vi "PH_Cam_BaseClass.set Cam Error.vi"(0 "VI in":refnum<vi>, 3 "Cam Error":errorcluster, 5 "error in":errorcluster) -> (14 "VI out":refnum<vi>, 19 "error out":errorcluster)   [LabVIEW 2014, in "PH_Cam_BaseClass.lvlib"]
doc: "This VI sets the Cam Error to own attributes and the GUI if it has changed."
uses:
  PH_Cam_BaseClass.lvlib
  PH_Common/PH_Common.lvlib
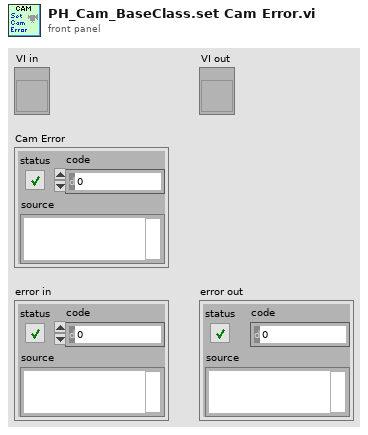
[diagram p1: front panel]
types:
  T1 = typedef "PH_Cam_BaseClass.lvlib/PH_Cam_BaseClass.i attribute.ctl" = cluster{"Gui Refs":T2, "Cam":cluster{"Source Notifier":refnum<notifier>, "Error":errorcluster, "Camera ID":string}, "Images":cluster{"Cam":T3, "Operation":T3, "PSDB":T3}, "Window Image":cluster{"Indicate Image":bool, "Window No.":i32, "Scale Facor":dbl, "Center Cross":bool, "Subtract Backgr":bool, "CoG":bool, "Color Palette":cluster{"Red":u8, "Green":u8, "Blue":u8}[], "Image On":bool}, "Default Prdc Int":i32, "Performance":cluster{"on":bool, "Timestamp Last Frame":i32}, "Histogram":cluster{"on":bool, "Mapping":bool}, "Save Image":cluster{"Save":bool, "File refnum":refnum<file>}, "Setting Service ID":i32, "Screen":cluster{"x-resolution":i16, "y-resolution":i16}, "On":bool, "Constructor finished":bool, "configured":bool}
  T2 = typedef "PH_Cam_BaseClass.lvlib/PH_Cam_BaseClass.GUI Refs.ctl" = cluster{"Frame Rate":refnum<vi>, "Get Frame Rate":refnum<vi>, "Show Image":refnum<vi>, "Get Histogram":refnum<vi>, "Mapping":refnum<vi>, "Histogram":refnum<vi>, "Center Cross":refnum<vi>, "Center of Gravity":refnum<vi>, "Scale Factor [%]":refnum<vi>, "Save Image":refnum<vi>, "Palette":refnum<vi>, "Subtract Background":refnum<vi>, "Cam Error":refnum<vi>, "On":refnum<vi>, "Cam List":refnum<vi>}
  T3 = typedef "IMAQ Image.ctl" = refnum<image>
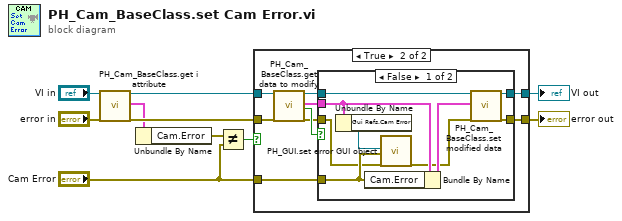
[diagram p0: block diagram]
diagram:
  n1 = call "PH_Cam_BaseClass.get i attribute.vi"("i ref in"="VI in", "error in (no error)"="error in") -> ("i ref out"=w7:refnum<vi>, "i attribute"=w4:T1, "error out"=w5:errorcluster)  [unwired: 15 in]
  n2 = Unbundle By Name(w4) -> ("Cam.Error"=w3:errorcluster)
  n3 = Not Equal?(x=w3, y="Cam Error") -> (x != y?=w1:bool)
  n4 = case shown="True" w1 {
    tunnel: [w11 w21] -> w10
    tunnel: [w12 w20] -> w8
    tunnel: w7 -> [w12 w15]
    tunnel: w5 -> [w11 w14]
    tunnel: "Cam Error" -> [_ w13]
    frame False {
    }
    frame True {
      n5 = call "PH_Cam_BaseClass.get data to modify.vi"("i ref in"=w15, "error in (no error)"=w14) -> ("i ref out"=w17:refnum<vi>, "i attribute"=w18:T1, "timed out"=w19:bool, "error out"=w16:errorcluster)  [unwired: 14 in]
      n6 = case shown="False" w19 {
        tunnel: w16 -> [w22 w31]
        tunnel: [w30 w31] -> w21
        tunnel: w17 -> [w29 w32]
        tunnel: [w28 w32] -> w20
        tunnel: w18 -> [w26 _]
        tunnel: w13 -> [w24 _]
        frame False {
          n7 = Unbundle By Name(w26) -> ("Gui Refs.Cam Error"=w23:refnum<vi>)
          n8 = Bundle By Name(cluster=w26, "Cam.Error"=w24) -> (w27:T1)
          n9 = call "PH_GUI.set error GUI object.vi"("GUI Refs.Device Error"=w23, "error to set"=w24, "error in (no error)"=w22) -> ("error out"=w25:errorcluster)  [unwired: 16 in]
          n10 = call "PH_Cam_BaseClass.set modified data.vi"("i ref in"=w29, "i attribute"=w27, "error in (no error)"=w25) -> ("i ref out"=w28:refnum<vi>, "error out"=w30:errorcluster)  [unwired: 15 in]
        }
        frame True {
        }
      }
    }
  }
  "error out" <- w10
  "VI out" <- w8
